vi "FPGA upload data to LEDs.vi"   [LabVIEW 2015]
uses:
  <vilib>/rvi/Emulation/niFpgaGetClockAttributes.vi
  <vilib>/rvi/Emulation/niFpgaSctlEmulationGetInTimedLoop.vi
  <vilib>/rvi/Emulation/niFpgaEmulationReportErrorSimple.vi
  <vilib>/rvi/DataTransferAndStorage/Container/Common/niFpgaContainerGetUniqueNameForEmu.vi
  <vilib>/rvi/DataTransferAndStorage/Container/Common/niFpgaContainerSetEmuInfo.vi
  <vilib>/rvi/eio/common/nirviEmuReportErrorAndStop.vi
  <vilib>/rvi/DataTransferAndStorage/Container/Common/niFpgaContainerExecOnDevCompGetState.vi
  <vilib>/rvi/Emulation/niFpgaEmulationIsFPGAContextNoSignature.vi
  <vilib>/rvi/errors/niFpgaSetErrorForExecOnDevCompSimple.vi
  <vilib>/rvi/FIFO/Fifo_Resource/nirvififoEmulationSetSize.vi
  <vilib>/rvi/FIFO/Fifo_Resource/nirviFifoEmulationQueueMgr.vi
  <instcachedir>/0/nirviFifoEmulationQueueMgr_E5CAEC123FF24DC58D834DCA3CDAA9B5.lvgen/nirviFifoEmulationQueueMgr_E5CAEC123FF24DC58D834DCA3CDAA9B5_002.vi
  <vilib>/rvi/FIFO/Fifo_Resource/nirvififoEmulationDetermineInputValidOut.vi
  <vilib>/rvi/FIFO/Fifo_Resource/nirvififoEmulationCreateLock.vi
  <vilib>/rvi/Emulation/niFpgaProcessEmulError.vi
  <vilib>/rvi/FIFO/Fifo_Resource/nirvififoEmulationObtainLock.vi
  <vilib>/rvi/FIFO/Fifo_Resource/nirvififoEmulationReleaseLock.vi
  <vilib>/rvi/occurrence/nirviWaitOnOccurrenceBase.vi
  <vilib>/rvi/errors/nirviReportUnexpectedCaseInternalError.vi
  <vilib>/rvi/errors/nirviReportUnexpectedCaseInternalError (U32).vi
  <vilib>/Utility/error.llb/Clear Errors.vi
  <vilib>/rvi/interface/RandomDataEmulation/niFpgaRandomDataHandleErrors.vi
  <vilib>/rvi/Emulation/niFpgaCriticalErrorInLSC.vi
  <vilib>/rvi/LocalResourceManager/LocalResourceManager.xnode
  <vilib>/rvi/DataTransferAndStorage/Container/XNode/niFpgaContainer.xnode
  <vilib>/rvi/FIFO/Fifo_Resource/niFpgaFifoEmulationRefIn.vi
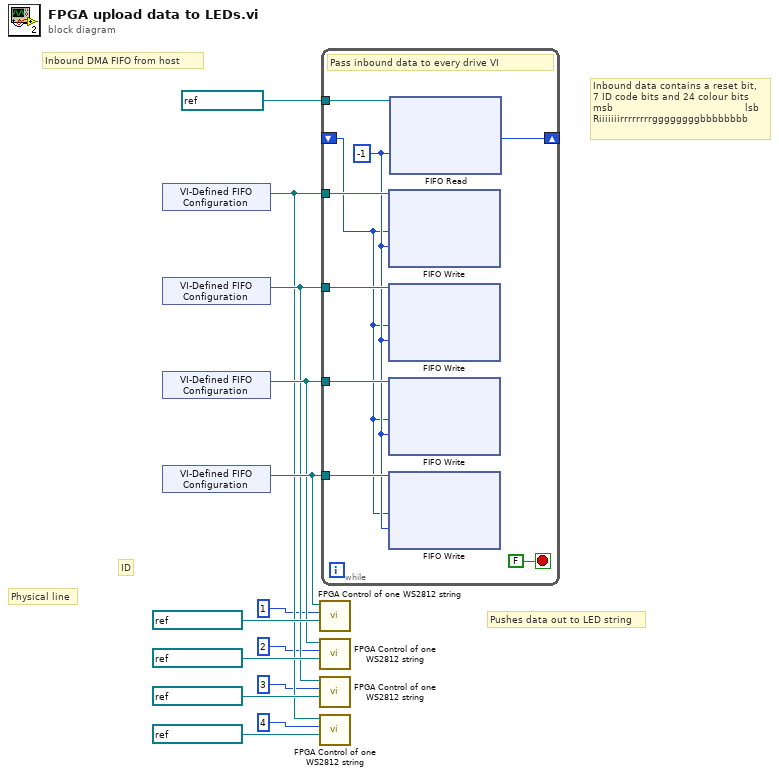
[diagram p0: block diagram]
diagram:
  # "Inbound DMA FIFO from host"
  # "Pushes data out to LED string"
  # "Physical line"
  # "ID"
  # "Inbound data contains a reset bit,\n7 ID code bits and 24 colour bits\nmsb                                            lsb\nRiiiiiiirrrrrrrrggggggggbbbbbbbb"
  n1 = xnode "VI-Defined FIFO Configuration"() -> ("FIFO Out"=w5:refnum<k21>)
  n2 = xnode "VI-Defined FIFO Configuration"() -> ("FIFO Out"=w6:refnum<k21>)
  n3 = xnode "VI-Defined FIFO Configuration"() -> ("FIFO Out"=w7:refnum<k21>)
  n4 = xnode "VI-Defined FIFO Configuration"() -> ("FIFO Out"=w8:refnum<k21>)
  n5 = call "FPGA Control of one WS2812 string.vi"("FPGA DO line"=refnum<k21> "Mod2/DIO0" ("FPGA I/O In"), "Wire ID"=u8 1 ("ID"), "FIFO In"=w8) -> ()  [unwired: 9 in]
  n6 = call "FPGA Control of one WS2812 string.vi"("FPGA DO line"=refnum<k21> "Mod2/DIO1" ("FPGA I/O In"), "Wire ID"=u8 2 ("ID"), "FIFO In"=w7) -> ()  [unwired: 9 in]
  n7 = call "FPGA Control of one WS2812 string.vi"("FPGA DO line"=refnum<k21> "Mod2/DIO2" ("FPGA I/O In"), "Wire ID"=u8 3 ("ID"), "FIFO In"=w6) -> ()  [unwired: 9 in]
  n8 = call "FPGA Control of one WS2812 string.vi"("FPGA DO line"=refnum<k21> "Mod2/DIO3" ("FPGA I/O In"), "Wire ID"=u8 4 ("ID"), "FIFO In"=w5) -> ()  [unwired: 9 in]
  n9 = while {
    tunnel: refnum<k21> "DMA FIFO" ("FIFO In") -> [w22]
    tunnel: w8 -> [w20]
    tunnel: w7 -> [w19]
    tunnel: w6 -> [w18]
    tunnel: w5 -> [w17]
    shift-right: [w15] -> _
    shift-left: _ -> [w14]
    stop <- FALSE stop-if-true
    w16 = -1 ("Timeout")
    # "Pass inbound data to every drive VI"
    n10 = xnode ("FIFO Write")("Element"=w14, "Timeout"=w16, "FIFO In"=w17) -> ()  [unwired: 2 out]
    n11 = xnode ("FIFO Write")("Element"=w14, "Timeout"=w16, "FIFO In"=w18) -> ()  [unwired: 2 out]
    n12 = xnode ("FIFO Write")("Element"=w14, "Timeout"=w16, "FIFO In"=w19) -> ()  [unwired: 2 out]
    n13 = xnode ("FIFO Write")("Element"=w14, "Timeout"=w16, "FIFO In"=w20) -> ()  [unwired: 2 out]
    n14 = xnode ("FIFO Read")("Timeout"=w16, "FIFO In"=w22) -> ("Element"=w15:u32)  [unwired: 2 out]
  }
